vi "CONNECT.checkValidID.vi"(8 "error in (no error)":errorcluster, 10 "CONNECT":refnum<class "CONNECT.lvclass">, 11 "Server in":refnum<class "Server.lvclass">) -> (0 "error out":errorcluster, 1 "valid ID":bool, 2 "client ID":string, 3 "Server out":refnum<class "Server.lvclass">)   [LabVIEW 2013, in "MQTT Server.lvlib" / "Server.lvclass"]
uses:
  Server.lvclass
  <vilib>/LabVIEW Open Source Project/MQTT Control Packets/Control Packets/CONNECT/CONNECT.lvclass
  <vilib>/LabVIEW Open Source Project/MQTT Control Packets/Control Packets/ControlPacket/ControlPacket.lvclass
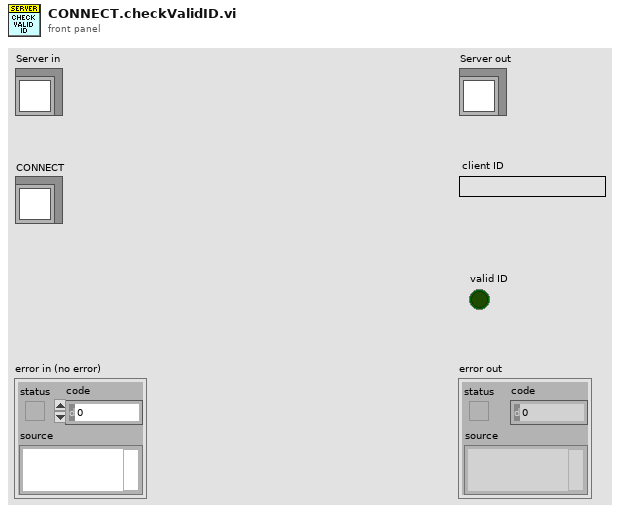
[diagram p1: front panel]
types:
  T1 = typedef "MQTT_Control_Packets.lvlib/CONNECT.lvclass/ConnectFlags -- cluster.ctl" = cluster{"Reserved":bool, "Clean Session":bool, "Will Flag":bool, "Will QoS 1":bool, "Will QoS 2":bool, "Will Retain":bool, "Password Flag":bool, "User Name Flag":bool}
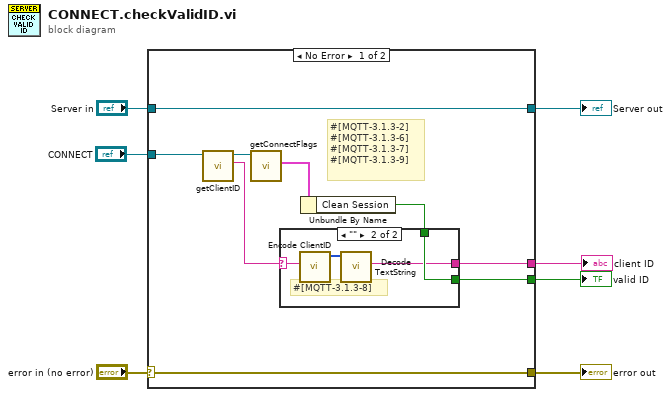
[diagram p0: block diagram]
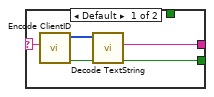
[diagram p2: hidden frame]
diagram:
  n1 = case shown="No Error" "error in (no error)" {
    selector: "error in (no error)" -> [w15 w26]
    tunnel: [w15 w26] -> w6
    tunnel: [w16 w25] -> w4
    tunnel: "Server in" -> [w16 w25]
    tunnel: "CONNECT" -> [w10 _]
    tunnel: [w9 _] -> w1
    tunnel: [w8 _] -> w2
    frame No Error {
      # "#[MQTT-3.1.3-2]\n#[MQTT-3.1.3-6]\n#[MQTT-3.1.3-7]\n#[MQTT-3.1.3-9]"
      n2 = call <vilib>:"getClientID.vi"("CONNECT in"=w10) -> ("Client ID"=w11:string, "CONNECT out"=w14:refnum<class "CONNECT.lvclass">)  [unwired: 9 in]
      n3 = call <vilib>:"getConnectFlags.vi"("CONNECT in"=w14) -> ("Connect Flags"=w13:T1)  [unwired: 9 in, 1 out]
      n4 = Unbundle By Name(w13) -> ("Clean Session"=w12:bool)
      n5 = case shown="\"\"" w11 {
        selector: w11 -> [w20 w23]
        tunnel: [w19 w24] -> w8
        tunnel: w12 -> [_ w24]
        tunnel: [w17 w21] -> w9
        frame Default {
          n6 = call <vilib>:"Encode ClientID.vi"("Client ID (empty: generate new)"=w20) -> ("valid Client ID"=w19:bool, "Length-Prefixed Field"=w18:u8[])  [unwired: 9 in]
          n7 = call <vilib>:"Decode TextString.vi"("Length-Prefixed Field"=w18) -> ("Text String"=w17:string)  [unwired: 8 in, 2 out]
        }
        frame "" {
          # "#[MQTT-3.1.3-8]"
          n8 = call <vilib>:"Encode ClientID.vi"("Client ID (empty: generate new)"=w23) -> ("Length-Prefixed Field"=w22:u8[])  [unwired: 9 in, 1 out]
          n9 = call <vilib>:"Decode TextString.vi"("Length-Prefixed Field"=w22) -> ("Text String"=w21:string)  [unwired: 8 in, 2 out]
        }
      }
    }
    frame Error {
    }
  }
  "error out" <- w6
  "Server out" <- w4
  "client ID" <- w1
  "valid ID" <- w2
